vi "array -- 3-finitediff.vi"(10 "ω (rad/sec)":cdb[](array[numeric])=[32012.991918577427+0.0i, 32390.261658505893+0.0i, 32466.39798177853+0.0i, 32499.14340521798+0.0i, 32517.39286113775+0.0i, 32529.046092051318+0.0i, 32537.14525712326+0.0i, 32543.111142615544+0.0i, 32547.696343954158+0.0i, 32551.33675949651+0.0i, 32554.302325209504+0.0i, 32556.769142360055+0.0i, 32558.856995237307+0.0i, 32560.650202739795+0.0i, 32562.209843476354+0.0i, 32563.58125099723+0.0i, 32564.7987833122+0.0i, 32565.88895894197+0.0i, 32566.872575330308+0.0i, 32567.766175404246+0.0i, 32568.583086316496+0.0i, 32569.334166794306+0.0i, 32570.02835688638+0.0i, 32570.673085530187+0.0i, 32571.274580490695+0.0i, 32571.838104118455+0.0i, 32572.36813539066+0.0i, 32572.868514009202+0.0i, 32573.342552524307+0.0i, 32573.793126289274+0.0i, 32574.222746575288+0.0i, 32574.633618125405+0.0i, 32575.027687968828+0.0i, 32575.40668442971+0.0i, 32575.772149741057+0.0i, 32576.12546690325+0.0i, 32576.467883345118+0.0i, 32576.800529469096+0.0i, 32577.124435064776+0.0i, 32577.440543590797+0.0i, 32577.749724325146+0.0i, 32578.052781957467+0.0i, 32578.35046682089+0.0i, 32578.643482565894+0.0i, 32578.932492128843+0.0i, 32579.218126471686+0.0i, 32579.500987779396+0.0i, 32579.781656707495+0.0i, 32580.06069600583+0.0i, 32580.338656060805+0.0i, 32580.616078519142+0.0i, 32580.89350097748+0.0i, 32581.171461032456+0.0i, 32581.45050033079+0.0i, 32581.73116925889+0.0i, 32582.0140305666+0.0i, 32582.29966469628+0.0i, 32582.58867447239+0.0i, 32582.88169000423+0.0i, 32583.179375080817+0.0i, 32583.48243271314+0.0i, 32583.791613234323+0.0i, 32584.10772197351+0.0i, 32584.43162756919+0.0i, 32584.764273480003+0.0i, 32585.106690135035+0.0i, 32585.460007297228+0.0i, 32585.825472395412+0.0i, 32586.204468856296+0.0i, 32586.59853891288+0.0i, 32587.009410462997+0.0i, 32587.439030535847+0.0i, 32587.889604513977+0.0i, 32588.363642815923+0.0i, 32588.86402143446+0.0i, 32589.39405291983+0.0i, 32589.957576334426+0.0i, 32590.559071508098+0.0i, 32591.203800151903+0.0i, 32591.897990030815+0.0i, 32592.64907072179+0.0i, 32593.46598163404+0.0i, 32594.359581707977+0.0i, 32595.343197883154+0.0i, 32596.433373726086+0.0i, 32597.650906041054+0.0i, 32599.022313348767+0.0i, 32600.58195429849+0.0i, 32602.375161800977+0.0i, 32604.46301467823+0.0i, 32606.929831615616+0.0i, 32609.895397541775+0.0i, 32613.535812870963+0.0i, 32618.12101442274+0.0i, 32624.086899701866+0.0i, 32632.186064986967+0.0i, 32643.839295900536+0.0i, 32662.088751820305+0.0i, 32694.834175046595+0.0i, 32770.97049853239+0.0i]) -> (2 "dω (rad/sec)":cdb[](array[numeric])=[32012.991918577427+0.0i, 32390.261658505893+0.0i, 32466.39798177853+0.0i, 32499.14340521798+0.0i, 32517.39286113775+0.0i, 32529.046092051318+0.0i, 32537.14525712326+0.0i, 32543.111142615544+0.0i, 32547.696343954158+0.0i, 32551.33675949651+0.0i, 32554.302325209504+0.0i, 32556.769142360055+0.0i, 32558.856995237307+0.0i, 32560.650202739795+0.0i, 32562.209843476354+0.0i, 32563.58125099723+0.0i, 32564.7987833122+0.0i, 32565.88895894197+0.0i, 32566.872575330308+0.0i, 32567.766175404246+0.0i, 32568.583086316496+0.0i, 32569.334166794306+0.0i, 32570.02835688638+0.0i, 32570.673085530187+0.0i, 32571.274580490695+0.0i, 32571.838104118455+0.0i, 32572.36813539066+0.0i, 32572.868514009202+0.0i, 32573.342552524307+0.0i, 32573.793126289274+0.0i, 32574.222746575288+0.0i, 32574.633618125405+0.0i, 32575.027687968828+0.0i, 32575.40668442971+0.0i, 32575.772149741057+0.0i, 32576.12546690325+0.0i, 32576.467883345118+0.0i, 32576.800529469096+0.0i, 32577.124435064776+0.0i, 32577.440543590797+0.0i, 32577.749724325146+0.0i, 32578.052781957467+0.0i, 32578.35046682089+0.0i, 32578.643482565894+0.0i, 32578.932492128843+0.0i, 32579.218126471686+0.0i, 32579.500987779396+0.0i, 32579.781656707495+0.0i, 32580.06069600583+0.0i, 32580.338656060805+0.0i, 32580.616078519142+0.0i, 32580.89350097748+0.0i, 32581.171461032456+0.0i, 32581.45050033079+0.0i, 32581.73116925889+0.0i, 32582.0140305666+0.0i, 32582.29966469628+0.0i, 32582.58867447239+0.0i, 32582.88169000423+0.0i, 32583.179375080817+0.0i, 32583.48243271314+0.0i, 32583.791613234323+0.0i, 32584.10772197351+0.0i, 32584.43162756919+0.0i, 32584.764273480003+0.0i, 32585.106690135035+0.0i, 32585.460007297228+0.0i, 32585.825472395412+0.0i, 32586.204468856296+0.0i, 32586.59853891288+0.0i, 32587.009410462997+0.0i, 32587.439030535847+0.0i, 32587.889604513977+0.0i, 32588.363642815923+0.0i, 32588.86402143446+0.0i, 32589.39405291983+0.0i, 32589.957576334426+0.0i, 32590.559071508098+0.0i, 32591.203800151903+0.0i, 32591.897990030815+0.0i, 32592.64907072179+0.0i, 32593.46598163404+0.0i, 32594.359581707977+0.0i, 32595.343197883154+0.0i, 32596.433373726086+0.0i, 32597.650906041054+0.0i, 32599.022313348767+0.0i, 32600.58195429849+0.0i, 32602.375161800977+0.0i, 32604.46301467823+0.0i, 32606.929831615616+0.0i, 32609.895397541775+0.0i, 32613.535812870963+0.0i, 32618.12101442274+0.0i, 32624.086899701866+0.0i, 32632.186064986967+0.0i, 32643.839295900536+0.0i, 32662.088751820305+0.0i, 32694.834175046595+0.0i, 32770.97049853239+0.0i])   [LabVIEW 2021]
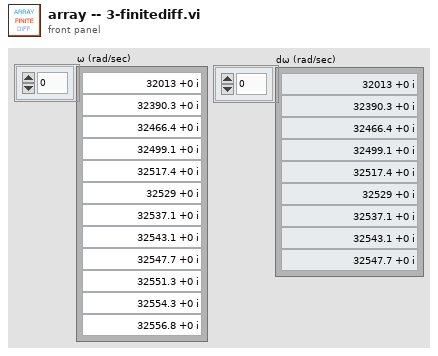
[diagram p1: front panel]
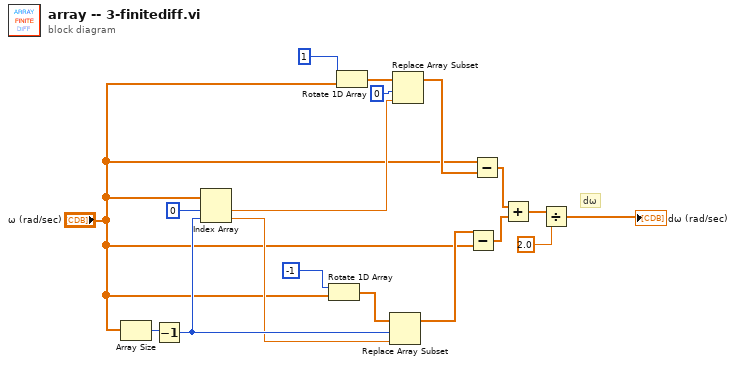
[diagram p0: block diagram]
diagram:
  # "dω"
  n1 = Array Size(array="ω (rad/sec)") -> (size(s)=w17:i32)
  n2 = Decrement(x=w17) -> (x-1=w10:i32)
  n3 = Index Array(array="ω (rad/sec)", index #1=0 ("index"), index #2=w10) -> (element #1=w13:cdb, element #2=w9:cdb)
  n4 = Rotate 1D Array(1:"ω (rad/sec)", 2:-1 ("n")) -> (0:w11:cdb[])
  n5 = Rotate 1D Array(1:"ω (rad/sec)", 2:1 ("n")) -> (0:w15:cdb[])
  n6 = Replace Array Subset(array=w11, new element=w9, index=w10) -> (w2:cdb[])
  n7 = Replace Array Subset(array=w15, new element=w13, index=0) -> (w3:cdb[])
  n8 = Subtract(x=w2, y="ω (rad/sec)") -> (x-y=w7:cdb[])
  n9 = Subtract(x="ω (rad/sec)", y=w3) -> (x-y=w8:cdb[])
  n10 = Add(x=w8, y=w7) -> (x+y=w6:cdb[])
  n11 = Divide(x=w6, y=2.0 ("n")) -> (x/y=→"dω (rad/sec)":cdb[])
